vi "shim_heater_get_state.vi"(8 "error in":errorcluster, 11 "conn_id_in":refnum<k5>) -> (0 "error out":errorcluster, 1 "ch2":bool, 2 "ch1":bool, 3 "conn_id_out":refnum<k5>, 4 "status":bool)   [LabVIEW 2019]
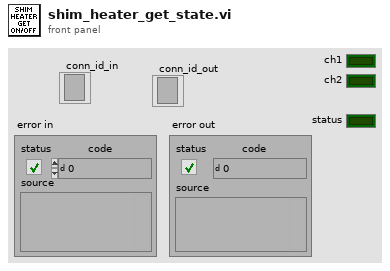
[diagram p1: front panel]
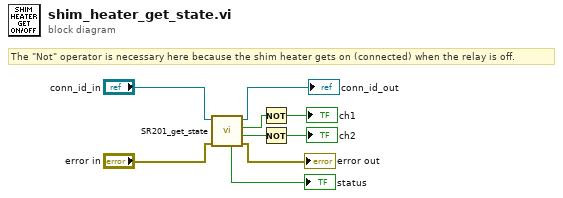
[diagram p0: block diagram]
diagram:
  # "The \"Not\" operator is necessary here because the shim heater gets on (connected) when the relay is off."
  n1 = call "SR201_get_state.vi"("error in"="error in", "conn_id_in"="conn_id_in") -> ("error out"=→"error out":errorcluster, "ch2"=w2:bool, "ch1"=w1:bool, "conn_id_out"=→"conn_id_out":refnum<k5>, "status"=→"status":bool)  [unwired: 4 in, 1 out]
  n2 = Not(x=w1) -> (.not. x?=→"ch1":bool)
  n3 = Not(x=w2) -> (.not. x?=→"ch2":bool)
